vi "Launch_gage_digitizer.vi"   [LabVIEW 2015]
uses:
  Pulse Echo Actor Project/Gage digitizer actor.lvclass
  <vilib>/ActorFramework/Actor/Actor.lvclass
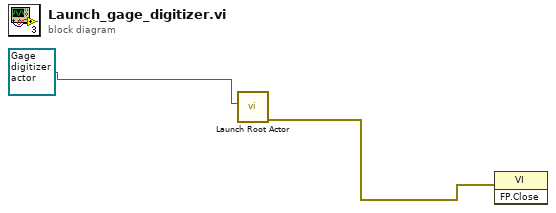
[diagram p0: block diagram]
diagram:
  n1 = call <vilib>:"Launch Root Actor.vi"("Actor"=refnum<class "Gage digitizer actor.lvclass"> refnum ("Gage digitizer actor.lvclass")) -> ("error out"=w2:errorcluster)  [unwired: 9 in, 1 out]
  n2 = invoke class="VI" method="FP.Close"(error in=w2) -> ()  [unwired: 2 in, 3 out]
